vi "niFPGA LM CU.vi"(9 "enable":bool, 10 "dataRDYIn":bool, 11 "reset":bool) -> (0 "dataReady?":bool, 1 "clear acc?":bool, 2 "coefIdx":u16, 3 "dataIdx":u16, 4 "idle?":bool, 5 "memWRAddr":u16)   [LabVIEW 2017]
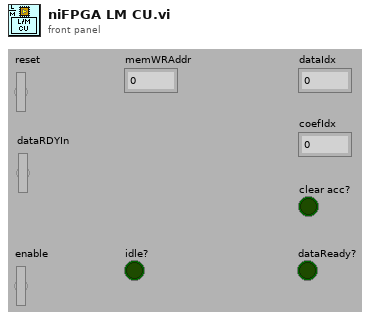
[diagram p1: front panel]
types:
  T1 = cluster{"kPhaseCnt":fxp<+,2,2>, "kMacCnt":fxp<+,7,7>, "kChanCntFiltering":fxp<+,1,1>, "kChanCntBuffer":fxp<+,1,1>, "kBufPtr":fxp<+,7,7>, "kCurrSample":fxp<+,7,7>, "kFutureLen":fxp<+,7,7>, "idle?":bool, "dataReady?":bool, "clear acc?":bool, "first run?":bool}
  T2 = cluster{"kTotalChan-1":fxp<+,1,1>, "kTapsPerPhase-1":fxp<+,6,6>, "kQ(floor(M/L))":fxp<+,1,1>, "kR(rem(M/L))":fxp<+,1,1>, "kL":fxp<+,2,2>, "kM":fxp<+,2,2>, "kBufSize":fxp<+,6,6>}
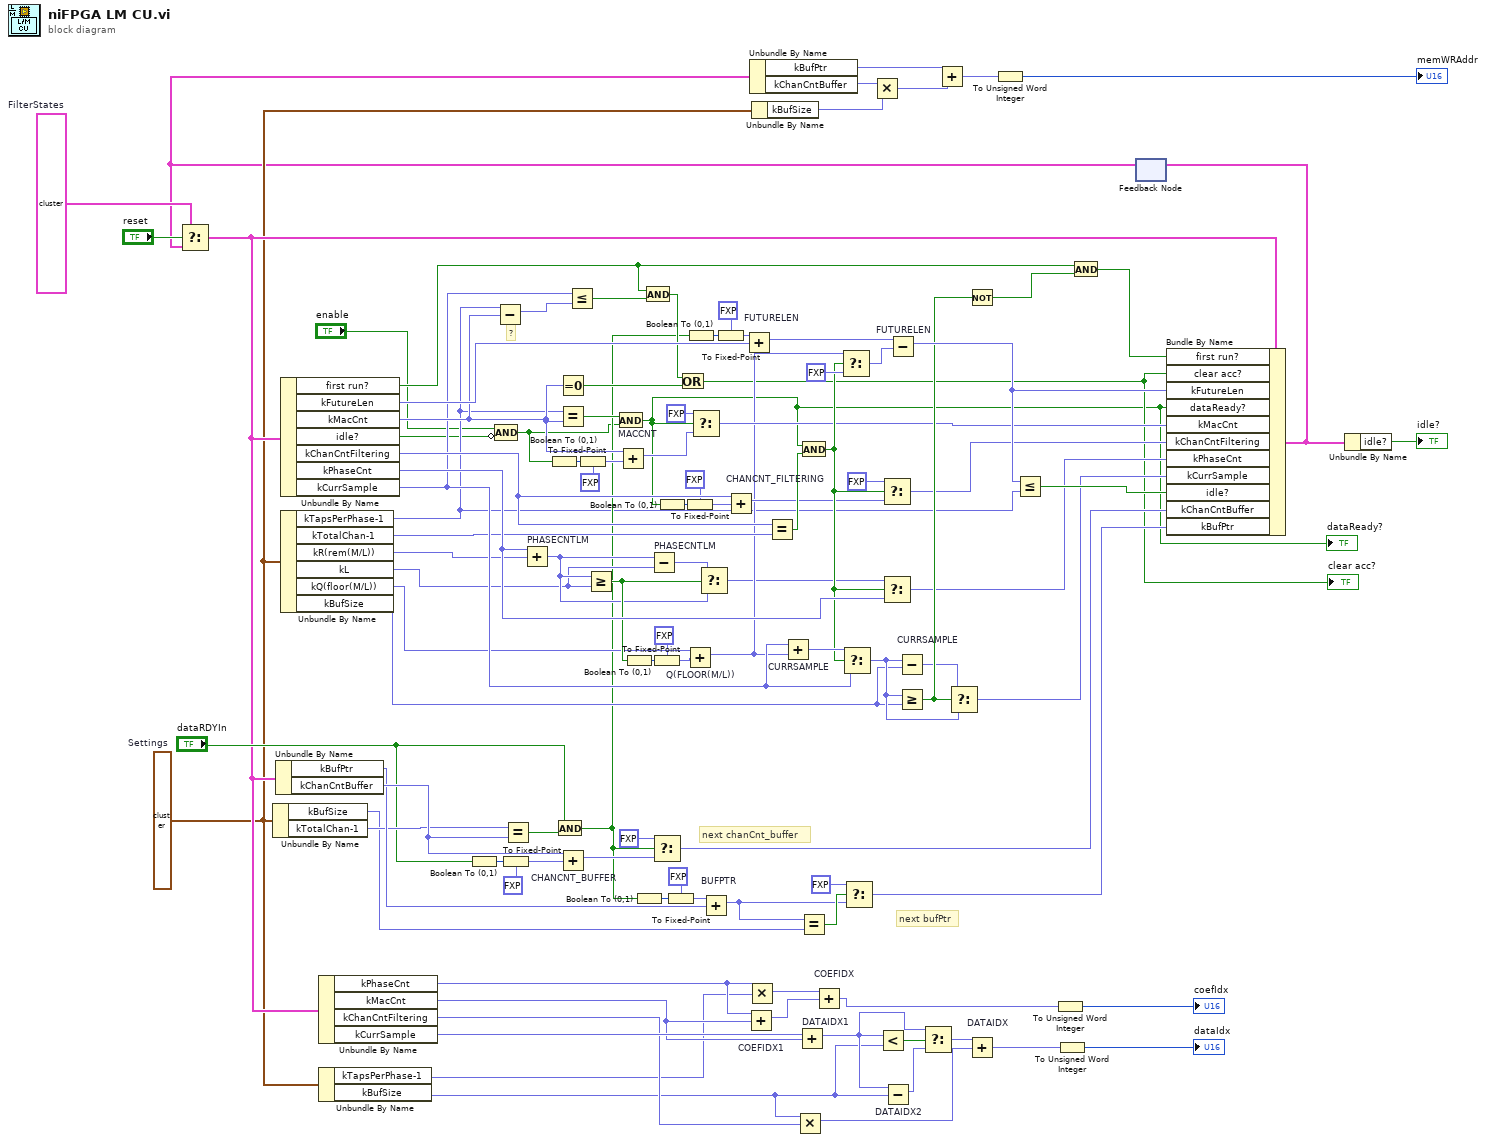
[diagram p0: block diagram]
diagram:
  w17 = T1 {"kPhaseCnt"=0.0, "kMacCnt"=0.0, "kChanCntFiltering"=0.0, "kChanCntBuffer"=0.0, "kBufPtr"=112.0, "kCurrSample"=0.0, "kFutureLen"=112.0, "idle?"=TRUE, "dataReady?"=FALSE, "clear acc?"=TRUE, "first run?"=TRUE}  # FilterStates
  w13 = T2 {"kTotalChan-1"=0.0, "kTapsPerPhase-1"=0.0, "kQ(floor(M/L))"=0.0, "kR(rem(M/L))"=0.0, "kL"=0.0, "kM"=0.0, "kBufSize"=0.0}  # Settings
  # "?"
  # "next bufPtr"
  # "next chanCnt_buffer"
  n1 = Unbundle By Name(w13) -> ("kBufSize"=w34:fxp<+,6,6>, "kTotalChan-1"=w35:fxp<+,1,1>)
  n2 = Unbundle By Name(w13) -> ("kTapsPerPhase-1"=w6:fxp<+,6,6>, "kTotalChan-1"=w67:fxp<+,1,1>, "kR(rem(M/L))"=w68:fxp<+,1,1>, "kL"=w69:fxp<+,2,2>, "kQ(floor(M/L))"=w70:fxp<+,1,1>, "kBufSize"=w71:fxp<+,6,6>)
  n3 = Unbundle By Name(w13) -> ("kTapsPerPhase-1"=w51:fxp<+,6,6>, "kBufSize"=w50:fxp<+,6,6>)
  n4 = Boolean To (0,1)(Boolean="dataRDYIn") -> (0, 1=w40:i16)
  n5 = To Fixed-Point(fixed-point type=fxp<+,1,1> 0.0 ("t"), number=w40) -> (fixed-point=w39:fxp<+,1,1>)
  n6 = Unbundle By Name(w13) -> ("kBufSize"=w12:fxp<+,6,6>)
  n7 = feedback #1() -> (w8:T1)  [unwired: 1 out]
  n8 = Select(t=w17, s="reset", f=w8) -> (s? t:f=w19:T1)
  n9 = Unbundle By Name(w19) -> ("kBufPtr"=w41:fxp<+,7,7>, "kChanCntBuffer"=w42:fxp<+,1,1>)
  n10 = Unbundle By Name(w19) -> ("first run?"=w87:bool, "kFutureLen"=w101:fxp<+,7,7>, "kMacCnt"=w84:fxp<+,7,7>, "idle?"=w3:bool, "kChanCntFiltering"=w93:fxp<+,1,1>, "kPhaseCnt"=w106:fxp<+,2,2>, "kCurrSample"=w78:fxp<+,7,7>)
  n11 = Unbundle By Name(w19) -> ("kPhaseCnt"=w53:fxp<+,2,2>, "kMacCnt"=w52:fxp<+,7,7>, "kChanCntFiltering"=w57:fxp<+,1,1>, "kCurrSample"=w61:fxp<+,7,7>)
  n12 = Subtract(x=w6, y=w84) -> (x-y=w83:fxp<+/-,8,8>)
  n13 = Compound Arithmetic op=AND("enable", invert w3) -> (w1:bool)
  n14 = Equal?(x=w35, y=w42) -> (x = y?=w36:bool)
  n15 = Add "PHASECNTLM"(x=w106, y=w68) -> (x+y=w79:fxp<+,2,2>)
  n16 = Boolean To (0,1)(Boolean=w1) -> (0, 1=w107:i16)
  n17 = And(x="dataRDYIn", y=w36) -> (x .and. y?=w7:bool)
  n18 = Equal To 0?(x=w84) -> (x = 0?=w95:bool)
  n19 = Equal?(x=w6, y=w84) -> (x = y?=w94:bool)
  n20 = Add "CHANCNT_BUFFER"(x=w42, y=w39) -> (x+y=w37:fxp<+,1,1>)
  n21 = Less Or Equal?(x=w78, y=w83) -> (x <= y?=w81:bool)
  n22 = To Fixed-Point(fixed-point type=fxp<+,1,1> 0.0, number=w107) -> (fixed-point=w108:fxp<+,1,1>)
  n23 = Greater Or Equal?(x=w79, y=w69) -> (x >= y?=w104:bool)
  n24 = And(x=w94, y=w1) -> (x .and. y?=w5:bool)
  "dataReady?" <- w5
  n25 = Add "MACCNT"(x=w84, y=w108) -> (x+y=w109:fxp<+,6,6>)
  n26 = Boolean To (0,1)(Boolean=w104) -> (0, 1=w105:i16)
  n27 = Boolean To (0,1)(Boolean=w7) -> (0, 1=w47:i16)
  n28 = And(x=w87, y=w81) -> (x .and. y?=w91:bool)
  n29 = Subtract "PHASECNTLM"(x=w79, y=w69) -> (x-y=w80:fxp<+,2,2>)
  n30 = To Fixed-Point(fixed-point type=fxp<+,1,1> 0.0 ("t"), number=w105) -> (fixed-point=w103:fxp<+,1,1>)
  n31 = Select(t=fxp<+,1,1> 0.0, s=w7, f=w37) -> (s? t:f=w32:fxp<+,1,1>)
  n32 = Boolean To (0,1)(Boolean=w5) -> (0, 1=w75:i16)
  n33 = To Fixed-Point(fixed-point type=fxp<+,1,1> 0.0 ("t"), number=w47) -> (fixed-point=w46:fxp<+,1,1>)
  n34 = Or(x=w91, y=w95) -> (x .or. y?=w9:bool)
  "clear acc?" <- w9
  n35 = To Fixed-Point(fixed-point type=fxp<+,1,1> 0.0, number=w75) -> (fixed-point=w74:fxp<+,1,1>)
  n36 = Add "Q(FLOOR(M/L))"(x=w70, y=w103) -> (x+y=w22:fxp<+,1,1>)
  n37 = Boolean To (0,1)(Boolean=w7) -> (0, 1=w102:i16)
  n38 = Select(t=fxp<+,1,1> 0.0, s=w5, f=w109) -> (s? t:f=w66:fxp<+,6,6>)
  n39 = Select(t=w80, s=w104, f=w79) -> (s? t:f=w21:fxp<+,2,2>)
  n40 = Add "BUFPTR"(x=w46, y=w41) -> (x+y=w44:fxp<+,6,6>)
  n41 = To Fixed-Point(fixed-point type=fxp<+,1,1> 0.0, number=w102) -> (fixed-point=w90:fxp<+,1,1>)
  n42 = Add "CHANCNT_FILTERING"(x=w93, y=w74) -> (x+y=w72:fxp<+,1,1>)
  n43 = Add "FUTURELEN"(x=w90, y=w101) -> (x+y=w99:fxp<+,6,6>)
  n44 = Add "COEFIDX1"(x=w53, y=w52) -> (x+y=w54:fxp<+,6,6>)
  n45 = Multiply(x=w53, y=w51) -> (x*y=w62:fxp<+,8,8>)
  n46 = Unbundle By Name(w8) -> ("kBufPtr"=w15:fxp<+,7,7>, "kChanCntBuffer"=w14:fxp<+,1,1>)
  n47 = Equal?(x=w93, y=w67) -> (x = y?=w82:bool)
  n48 = Add "CURRSAMPLE"(x=w78, y=w22) -> (x+y=w100:fxp<+,6,6>)
  n49 = Multiply(x=w50, y=w57) -> (x*y=w55:fxp<+,6,6>)
  n50 = Add "DATAIDX1"(x=w61, y=w52) -> (x+y=w59:fxp<+,6,6>)
  n51 = And(x=w5, y=w82) -> (x .and. y?=w92:bool)
  n52 = Equal?(x=w44, y=w34) -> (x = y?=w45:bool)
  n53 = Add "COEFIDX"(x=w62, y=w54) -> (x+y=w48:fxp<+,8,8>)
  n54 = Select(t=w22, s=w92, f=fxp<+,1,1> 0.0) -> (s? t:f=w97:fxp<+,1,1>)
  n55 = Select(t=w100, s=w92, f=w78) -> (s? t:f=w76:fxp<+,7,7>)
  n56 = Select(t=fxp<+,1,1> 0.0, s=w45, f=w44) -> (s? t:f=w31:fxp<+,6,6>)
  n57 = Multiply(x=w14, y=w12) -> (x*y=w16:fxp<+,6,6>)
  n58 = Less?(x=w59, y=w50) -> (x < y?=w60:bool)
  n59 = Select(t=fxp<+,1,1> 0.0, s=w92, f=w72) -> (s? t:f=w65:fxp<+,1,1>)
  n60 = Select(t=w21, s=w92, f=w106) -> (s? t:f=w64:fxp<+,2,2>)
  n61 = Subtract "DATAIDX2"(x=w59, y=w50) -> (x-y=w58:fxp<+,6,6>)
  n62 = Subtract "FUTURELEN"(x=w99, y=w97) -> (x-y=w89:fxp<+,6,6>)
  n63 = Subtract "CURRSAMPLE"(x=w76, y=w71) -> (x-y=w77:fxp<+,6,6>)
  n64 = Greater Or Equal?(x=w76, y=w71) -> (x >= y?=w85:bool)
  n65 = Select(t=w59, s=w60, f=w58) -> (s? t:f=w56:fxp<+,6,6>)
  n66 = Add(x=w15, y=w16) -> (x+y=w11:fxp<+,8,8>)
  n67 = Select(t=w77, s=w85, f=w76) -> (s? t:f=w63:fxp<+,7,7>)
  n68 = Not(x=w85) -> (.not. x?=w86:bool)
  n69 = Add "DATAIDX"(x=w56, y=w55) -> (x+y=w49:fxp<+,6,6>)
  n70 = To Unsigned Word Integer(number=w11) -> (unsigned 16bit integer=→"memWRAddr":u16)
  n71 = Less Or Equal?(x=w89, y=w6) -> (x <= y?=w96:bool)
  n72 = To Unsigned Word Integer(number=w48) -> (unsigned 16bit integer=→"coefIdx":u16)
  n73 = To Unsigned Word Integer(number=w49) -> (unsigned 16bit integer=→"dataIdx":u16)
  n74 = And(x=w87, y=w86) -> (x .and. y?=w88:bool)
  n75 = Bundle By Name(cluster=w19, "first run?"=w88, "clear acc?"=w9, "kFutureLen"=w89, "dataReady?"=w5, "kMacCnt"=w66, "kChanCntFiltering"=w65, "kPhaseCnt"=w64, "kCurrSample"=w63, "idle?"=w96, "kChanCntBuffer"=w32, "kBufPtr"=w31) -> (w4:T1)
  n76 = feedback-in #1(w4) -> ()
  n77 = Unbundle By Name(w4) -> ("idle?"=→"idle?":bool)
